vi "Lab Panel V4.85.vi"() -> ()   [LabVIEW 2013] (continued)
                    # "start new test and create test file"
                    n881 = stacked-sequence {
                      seq-local: [w1542 _ _ _ _] -> [_ w1566 _ _ _]
                      tunnel: w1541 -> [w1547 _ _ _ _]
                      tunnel: w1540 -> [w1543 _ _ _ _]
                      tunnel: w1539 -> [w1557 _ _ _ _]
                      tunnel: w1538 -> [w1550 _ _ _ _]
                      tunnel: w1537 -> [w1545 _ _ _ _]
                      tunnel: [_ w1561 _ _ _] -> w1536
                      tunnel: w1535 -> [_ _ _ w1586 _]
                      tunnel: w1534 -> [_ _ _ w1585 _]
                      tunnel: w1533 -> [_ _ _ w1584 _]
                      frame #0 {
                        w1544 = "\\"
                        n882 = local read "SET LAB05-1"() -> (w1552:T5)
                        n883 = case shown="\"CYCLE TEST\"" w1557 {
                          tunnel: ["L05-1-CHART TEST-" "L05-1-CYCLE TEST-" "L05-1-T-RISE TEST-"] -> w1553
                          frame "CHART TEST", Default {
                          }
                          frame "CYCLE TEST" {
                          }
                          frame "T-RISE TEST" {
                          }
                        }
                        n884 = Unbundle(w1552) -> ("DESCRIPTION"=w1551:string)  [unwired: 4 out]
                        n885 = Concatenate Strings(w1547, "\\", w1545, w1544, w1543, w1544) -> (w1554:string)
                        n886 = String To Path(string=w1554) -> (path=w1556:path)
                        n887 = Concatenate Strings(w1554, w1553, w1551, "-", w1550, ".tdms") -> (w1542:string)
                        n888 = Create Folder(path (use dialog)=w1556) -> (error out=w1555:errorcluster)  [unwired: 2 in, 2 out]
                        n889 = global write "Global 1.vi" "LAB05-1 FILE"(w1542) -> ()
                        n890 = call <vilib>:"Clear Errors.vi"("error in (no error)"=w1555) -> ()  [unwired: 6 in, 1 out]
                      }
                      frame #1 {
                        (unwired) FALSE
                        n891 = String To Path(string=w1566) -> (path=w1562:path)
                        n892 = TDMS Open(6:FALSE, 10:T18."create or replace" ("operation (0:open)"), 11:w1562) -> (0:w1561:errorcluster, 3:→"TDMS LAB05-1":refnum<k34>)  [unwired: 4 in]
                      }
                      frame #2 {
                        n893 = local read "SET LAB05-1"() -> (w1572:T5)
                        n894 = local read "TDMS LAB05-1"() -> (w1583:refnum<k34>)
                        n895 = Build Array("Testers Name", "Description", "Set Test Cycles", "T-Rise minutes", "T-Rise Deg C") -> (w1573:string[])
                        n896 = Unbundle(w1572) -> ("NAME"=w1571:string, "DESCRIPTION"=w1570:string, "CYCLES"=w1569:dbl, "T-RISE mins"=w1568:dbl, "T-RISE deg C"=w1567:dbl)
                        n897 = Number To Decimal String(number=w1569) -> (decimal integer string=w1582:string)  [unwired: 1 in]
                        n898 = Number To Decimal String(number=w1568) -> (decimal integer string=w1581:string)  [unwired: 1 in]
                        n899 = Number To Decimal String(number=w1567) -> (decimal integer string=w1580:string)  [unwired: 1 in]
                        n900 = Build Array(w1571, w1570, w1582, w1581, w1580) -> (w1579:string[])
                        n901 = TDMS Set Properties(5:w1579, 7:w1573, 11:w1583) -> ()  [unwired: 3 in, 4 out]
                      }
                      frame #3 {
                        n902 = local read "DISP LAB05-1"() -> (w1588:T4)
                        n903 = Concatenate Strings("LAB05-1  ", w1586) -> (w1589:string)
                        n904 = Two Button Dialog(message=w1589, 1:w1584, 2:w1585) -> (T button?=w1591:bool)
                        n905 = case shown="True" w1591 {
                          tunnel: w1588 -> [w1598 w1599]
                          tunnel: [w1598 w1599] -> w1595
                          tunnel: [w1597 w1600] -> w1594
                          tunnel: [w1596 w1600] -> w1593
                          frame False {
                            n906 = Unbundle(w1598) -> ("CYCLE"=w1597:dbl, "MINS"=w1596:dbl)  [unwired: 1 out]
                          }
                          frame True {
                            w1600 = 0.0
                          }
                        }
                        n907 = Bundle(cluster=w1595, "CYCLE"=w1594, "MINS"=w1593, "STATUS"="RUN") -> (w1587:T4)
                        n908 = local write "DISP LAB05-1"(w1587) -> ()
                      }
                      frame #4 {
                        n909 = local read "SIG LAB05-1"() -> (w1603:T2)
                        n910 = local read "TEMP START LAB05-1"() -> (w1605:cluster{"TL":dbl, "TN":dbl})
                        n911 = Unbundle(w1603) -> ("Tmp Live"=w1602:dbl, "Tmp Neut"=w1601:dbl)  [unwired: 3 out]
                        n912 = Bundle(cluster=w1605, "TL"=w1602, "TN"=w1601) -> (w1604:cluster{"TL":dbl, "TN":dbl})
                        n913 = local write "TEMP START LAB05-1"(w1604) -> ()
                      }
                    }
                  }
                }
              }
              event "RUN LAB05-2": Value Change {
                n914 = event-data() -> ("NewVal"=w1609:bool)  [unwired: 1 in, 5 out]
                n915 = local write "run lab05-2"(w1609) -> ()
                n916 = case shown="True" w1609 {
                  tunnel: w1615 -> [_ w1651]
                  tunnel: w1614 -> [_ w1650]
                  tunnel: w1612 -> [w1617 w1649]
                  tunnel: w1613 -> [_ w1648]
                  tunnel: w1611 -> [_ w1647]
                  tunnel: [w1616 w1646] -> w1610
                  tunnel: w1608 -> [_ w1645]
                  tunnel: w1607 -> [_ w1644]
                  tunnel: w1606 -> [_ w1643]
                  frame False {
                    # "stop test"
                    n917 = stacked-sequence {
                      tunnel: w1617 -> [w1626 _]
                      tunnel: [w1618 _] -> w1616
                      frame #0 {
                        n918 = local read "DISP LAB05-2"() -> (w1625:T4)
                        n919 = Unbundle(w1625) -> ("CYCLE"=w1623:dbl, "MINS"=w1624:dbl)  [unwired: 1 out]
                        n920 = case shown="\"CYCLE TEST\"" w1626 {
                          tunnel: w1624 -> [_ _ w1633]
                          tunnel: w1623 -> [w1631 w1632 _]
                          tunnel: [w1631 w1632 w1633] -> w1622
                          frame "CHART TEST", Default {
                          }
                          frame "CYCLE TEST" {
                          }
                          frame "T-RISE TEST" {
                          }
                        }
                        n921 = local read "TDMS LAB05-2"() -> (w1630:refnum<k34>)
                        n922 = Build Array("STOPPED") -> (w1627:string[])
                        n923 = Build Array(w1622) -> (w1621:dbl[])
                        n924 = TDMS Write(0:w1630, 5:"TEST RESULT", 7:w1627, 9:w1621) -> (4:w1619:refnum<k34>, 15:w1620:errorcluster)  [unwired: 2 in, 2 out]
                        n925 = TDMS Close(8:w1620, 11:w1619) -> (0:w1618:errorcluster)  [unwired: 1 out]
                      }
                      frame #1 {
                        n926 = local read "DISP LAB05-2"() -> (w1637:T4)
                        n927 = stacked-sequence {
                          tunnel: "LAB05-2" -> [w1639 w1641]
                          frame #0 {
                            n928 = call "sub vi - defrag tdms v1.vi"("panel id"=w1639) -> ("error out"=w1638:errorcluster)  [unwired: 10 in]
                            n929 = local write "data file error"(w1638) -> ()
                          }
                          frame #1 {
                            n930 = local write "RESULT LAB05-2"(FALSE) -> ()
                            n931 = call "Save data file to network drive v2.vi"("panel id"=w1641) -> ("network file save error"=w1640:errorcluster)  [unwired: 9 in, 1 out]
                            n932 = local write "data file error"(w1640) -> ()
                          }
                        }
                        n933 = Bundle(cluster=w1637, "STATUS"="STOP") -> (w1635:T4)  [unwired: 2 in]
                        n934 = local write "DISP LAB05-2"(w1635) -> ()
                      }
                    }
                  }
                  frame True {
                    # "start new test and create test file"
                    n935 = stacked-sequence {
                      seq-local: [w1652 _ _ _ _] -> [_ w1676 _ _ _]
                      tunnel: w1651 -> [w1657 _ _ _ _]
                      tunnel: w1650 -> [w1653 _ _ _ _]
                      tunnel: w1649 -> [w1667 _ _ _ _]
                      tunnel: w1648 -> [w1660 _ _ _ _]
                      tunnel: w1647 -> [w1655 _ _ _ _]
                      tunnel: [_ w1671 _ _ _] -> w1646
                      tunnel: w1645 -> [_ _ _ w1696 _]
                      tunnel: w1644 -> [_ _ _ w1695 _]
                      tunnel: w1643 -> [_ _ _ w1694 _]
                      frame #0 {
                        w1654 = "\\"
                        n936 = local read "SET LAB05-2"() -> (w1662:T5)
                        n937 = case shown="\"CYCLE TEST\"" w1667 {
                          tunnel: ["L05-2-CHART TEST-" "L05-2-CYCLE TEST-" "L05-2-T-RISE TEST-"] -> w1663
                          frame "CHART TEST", Default {
                          }
                          frame "CYCLE TEST" {
                          }
                          frame "T-RISE TEST" {
                          }
                        }
                        n938 = Unbundle(w1662) -> ("DESCRIPTION"=w1661:string)  [unwired: 4 out]
                        n939 = Concatenate Strings(w1657, "\\", w1655, w1654, w1653, w1654) -> (w1664:string)
                        n940 = String To Path(string=w1664) -> (path=w1666:path)
                        n941 = Concatenate Strings(w1664, w1663, w1661, "-", w1660, ".tdms") -> (w1652:string)
                        n942 = Create Folder(path (use dialog)=w1666) -> (error out=w1665:errorcluster)  [unwired: 2 in, 2 out]
                        n943 = global write "Global 1.vi" "LAB05-2 FILE"(w1652) -> ()
                        n944 = call <vilib>:"Clear Errors.vi"("error in (no error)"=w1665) -> ()  [unwired: 6 in, 1 out]
                      }
                      frame #1 {
                        (unwired) FALSE
                        n945 = String To Path(string=w1676) -> (path=w1672:path)
                        n946 = TDMS Open(6:FALSE, 10:T18."create or replace" ("operation (0:open)"), 11:w1672) -> (0:w1671:errorcluster, 3:→"TDMS LAB05-2":refnum<k34>)  [unwired: 4 in]
                      }
                      frame #2 {
                        n947 = local read "SET LAB05-2"() -> (w1682:T5)
                        n948 = local read "TDMS LAB05-2"() -> (w1693:refnum<k34>)
                        n949 = Build Array("Testers Name", "Description", "Set Test Cycles", "T-Rise minutes", "T-Rise Deg C") -> (w1683:string[])
                        n950 = Unbundle(w1682) -> ("NAME"=w1681:string, "DESCRIPTION"=w1680:string, "CYCLES"=w1679:dbl, "T-RISE mins"=w1678:dbl, "T-RISE deg C"=w1677:dbl)
                        n951 = Number To Decimal String(number=w1679) -> (decimal integer string=w1692:string)  [unwired: 1 in]
                        n952 = Number To Decimal String(number=w1678) -> (decimal integer string=w1691:string)  [unwired: 1 in]
                        n953 = Number To Decimal String(number=w1677) -> (decimal integer string=w1690:string)  [unwired: 1 in]
                        n954 = Build Array(w1681, w1680, w1692, w1691, w1690) -> (w1689:string[])
                        n955 = TDMS Set Properties(5:w1689, 7:w1683, 11:w1693) -> ()  [unwired: 3 in, 4 out]
                      }
                      frame #3 {
                        n956 = local read "DISP LAB05-2"() -> (w1698:T4)
                        n957 = Concatenate Strings("LAB05-2  ", w1696) -> (w1699:string)
                        n958 = Two Button Dialog(message=w1699, 1:w1694, 2:w1695) -> (T button?=w1701:bool)
                        n959 = case shown="True" w1701 {
                          tunnel: w1698 -> [w1708 w1709]
                          tunnel: [w1708 w1709] -> w1705
                          tunnel: [w1707 w1710] -> w1704
                          tunnel: [w1706 w1710] -> w1703
                          frame False {
                            n960 = Unbundle(w1708) -> ("CYCLE"=w1707:dbl, "MINS"=w1706:dbl)  [unwired: 1 out]
                          }
                          frame True {
                            w1710 = 0.0
                          }
                        }
                        n961 = Bundle(cluster=w1705, "CYCLE"=w1704, "MINS"=w1703, "STATUS"="RUN") -> (w1697:T4)
                        n962 = local write "DISP LAB05-2"(w1697) -> ()
                      }
                      frame #4 {
                        n963 = local read "SIG LAB05-2"() -> (w1713:T2)
                        n964 = local read "TEMP START LAB05-2"() -> (w1715:cluster{"TL":dbl, "TN":dbl})
                        n965 = Unbundle(w1713) -> ("Tmp Live"=w1712:dbl, "Tmp Neut"=w1711:dbl)  [unwired: 3 out]
                        n966 = Bundle(cluster=w1715, "TL"=w1712, "TN"=w1711) -> (w1714:cluster{"TL":dbl, "TN":dbl})
                        n967 = local write "TEMP START LAB05-2"(w1714) -> ()
                      }
                    }
                  }
                }
              }
            }
            n968 = local write "data file error"(w587) -> ()
          }
          frame #4 {
            # "check if test cycles reached for cycle tests, if so then test pass"
            n969 = stacked-sequence {
              tunnel: w1735 -> [_ _ _ _ _ _ _ _ _ _]
              tunnel: w1734 -> [_ _ _ _ _ _ _ _ _ _]
              tunnel: w1733 -> [_ _ _ _ _ _ _ _ _ _]
              tunnel: w1732 -> [_ _ _ _ _ _ _ _ _ _]
              tunnel: w1731 -> [_ _ _ _ _ _ _ _ _ _]
              tunnel: w1730 -> [_ _ _ _ _ _ _ _ _ _]
              tunnel: w1729 -> [_ _ _ _ _ _ _ _ _ _]
              tunnel: w1728 -> [_ _ _ _ _ _ _ _ _ _]
              tunnel: w1727 -> [_ _ _ _ _ _ _ _ _ _]
              tunnel: w1726 -> [_ _ _ _ _ _ _ _ _ _]
              tunnel: w1725 -> [w1741 _ _ _ _ _ _ _ _ _]
              tunnel: w1724 -> [_ w1776 _ _ _ _ _ _ _ _]
              tunnel: w1723 -> [_ _ w1816 _ _ _ _ _ _ _]
              tunnel: w1722 -> [_ _ _ w1856 _ _ _ _ _ _]
              tunnel: w1721 -> [_ _ _ _ w1896 _ _ _ _ _]
              tunnel: w1720 -> [_ _ _ _ _ w1936 _ _ _ _]
              tunnel: w1719 -> [_ _ _ _ _ _ w1976 _ _ _]
              tunnel: w1718 -> [_ _ _ _ _ _ _ w2016 _ _]
              tunnel: w1717 -> [_ _ _ _ _ _ _ _ w2056 _]
              tunnel: w1716 -> [_ _ _ _ _ _ _ _ _ w2096]
              frame #0 {
                # "LAB01-1"
                n970 = Less?(x=w1741, y=2) -> (x < y?=w1739:bool)
                n971 = local read "DISP LAB01-1"() -> (w1742:T4)
                n972 = Unbundle(w1742) -> ("STATUS"=w1736:string)  [unwired: 2 out]
                n973 = Equal?(x=w1736, y="RUN") -> (x = y?=w1738:bool)
                n974 = And(x=w1738, y=w1739) -> (x .and. y?=w1737:bool)
                n975 = case shown="True" w1737 {
                  tunnel: w1742 -> [_ w1747]
                  tunnel: w1741 -> [_ w1751]
                  frame False {
                  }
                  frame True {
                    n976 = local read "SET LAB01-1"() -> (w1753:T5)
                    n977 = local read "TDMS LAB01-1"() -> (w1746:refnum<k34>)
                    n978 = Unbundle(w1753) -> ("CYCLES"=w1744:dbl, "T-RISE mins"=w1750:dbl)  [unwired: 3 out]
                    n979 = case shown="\"CYCLE TEST\"" w1751 {
                      tunnel: w1750 -> [_ _ w1760]
                      tunnel: [w1755 w1757 w1760] -> w1749
                      tunnel: w1744 -> [w1755 w1757 _]
                      tunnel: ["CHART PASS" "CYCLE PASS" "T-RISE PASS"] -> w1748
                      frame "CHART TEST", Default {
                      }
                      frame "CYCLE TEST" {
                      }
                      frame "T-RISE TEST" {
                      }
                    }
                    n980 = Unbundle(w1747) -> ("CYCLE"=w1752:dbl)  [unwired: 2 out]
                    n981 = Increment(x=w1744) -> (x+1=w1745:dbl)
                    n982 = Greater Or Equal?(x=w1752, y=w1745) -> (x >= y?=w1754:bool)
                    n983 = case shown="True" w1754 {
                      tunnel: w1749 -> [w1764 _]
                      tunnel: w1748 -> [w1763 _]
                      tunnel: w1747 -> [w1762 _]
                      tunnel: w1746 -> [w1761 _]
                      frame True {
                        n984 = stacked-sequence {
                          tunnel: w1764 -> [w1768 _]
                          tunnel: w1763 -> [w1766 w1772]
                          tunnel: w1762 -> [_ w1775]
                          tunnel: w1761 -> [w1765 _]
                          frame #0 {
                            n985 = Build Array(w1766) -> (w1769:string[])
                            n986 = Build Array(w1768) -> (w1767:dbl[])
                            n987 = TDMS Write(0:w1765, 5:"TEST PASS", 7:w1769, 9:w1767) -> (15:w1771:errorcluster)  [unwired: 2 in, 3 out]
                            n988 = local write "data file error"(w1771) -> ()
                          }
                          frame #1 {
                            n989 = Bundle(cluster=w1775, "STATUS"=w1772) -> (w1773:T4)  [unwired: 2 in]
                            n990 = local write "RESULT LAB01-1"(TRUE) -> ()
                            n991 = local write "DISP LAB01-1"(w1773) -> ()
                          }
                        }
                      }
                      frame False {
                      }
                    }
                  }
                }
              }
              frame #1 {
                # "LAB01-2"
                n992 = Less?(x=w1776, y=2) -> (x < y?=w1779:bool)
                n993 = local read "DISP LAB01-2"() -> (w1781:T4)
                n994 = Unbundle(w1781) -> ("STATUS"=w1782:string)  [unwired: 2 out]
                n995 = Equal?(x=w1782, y="RUN") -> (x = y?=w1778:bool)
                n996 = And(x=w1778, y=w1779) -> (x .and. y?=w1777:bool)
                n997 = case shown="True" w1777 {
                  tunnel: w1781 -> [_ w1787]
                  tunnel: w1776 -> [_ w1791]
                  frame False {
                  }
                  frame True {
                    n998 = local read "SET LAB01-2"() -> (w1793:T5)
                    n999 = local read "TDMS LAB01-2"() -> (w1786:refnum<k34>)
                    n1000 = Unbundle(w1793) -> ("CYCLES"=w1784:dbl, "T-RISE mins"=w1790:dbl)  [unwired: 3 out]
                    n1001 = case shown="\"T-RISE TEST\"" w1791 {
                      tunnel: w1790 -> [_ _ w1800]
                      tunnel: [w1795 w1797 w1800] -> w1789
                      tunnel: w1784 -> [w1795 w1797 _]
                      tunnel: ["CHART PASS" "CYCLE PASS" "T-RISE PASS"] -> w1788
                      frame "CHART TEST", Default {
                      }
                      frame "CYCLE TEST" {
                      }
                      frame "T-RISE TEST" {
                      }
                    }
                    n1002 = Unbundle(w1787) -> ("CYCLE"=w1792:dbl)  [unwired: 2 out]
                    n1003 = Increment(x=w1784) -> (x+1=w1785:dbl)
                    n1004 = Greater Or Equal?(x=w1792, y=w1785) -> (x >= y?=w1794:bool)
                    n1005 = case shown="True" w1794 {
                      tunnel: w1789 -> [w1804 _]
                      tunnel: w1788 -> [w1803 _]
                      tunnel: w1787 -> [w1802 _]
                      tunnel: w1786 -> [w1801 _]
                      frame True {
                        n1006 = stacked-sequence {
                          tunnel: w1804 -> [w1808 _]
                          tunnel: w1803 -> [w1806 w1812]
                          tunnel: w1802 -> [_ w1815]
                          tunnel: w1801 -> [w1805 _]
                          frame #0 {
                            n1007 = Build Array(w1806) -> (w1809:string[])
                            n1008 = Build Array(w1808) -> (w1807:dbl[])
                            n1009 = TDMS Write(0:w1805, 5:"TEST PASS", 7:w1809, 9:w1807) -> (15:w1811:errorcluster)  [unwired: 2 in, 3 out]
                            n1010 = local write "data file error"(w1811) -> ()
                          }
                          frame #1 {
                            n1011 = Bundle(cluster=w1815, "STATUS"=w1812) -> (w1813:T4)  [unwired: 2 in]
                            n1012 = local write "RESULT LAB01-2"(TRUE) -> ()
                            n1013 = local write "DISP LAB01-2"(w1813) -> ()
                          }
                        }
                      }
                      frame False {
                      }
                    }
                  }
                }
              }
              frame #2 {
                # "LAB02-1"
                n1014 = Less?(x=w1816, y=2) -> (x < y?=w1819:bool)
                n1015 = local read "DISP LAB02-1"() -> (w1821:T4)
                n1016 = Unbundle(w1821) -> ("STATUS"=w1822:string)  [unwired: 2 out]
                n1017 = Equal?(x=w1822, y="RUN") -> (x = y?=w1818:bool)
                n1018 = And(x=w1818, y=w1819) -> (x .and. y?=w1817:bool)
                n1019 = case shown="True" w1817 {
                  tunnel: w1821 -> [_ w1827]
                  tunnel: w1816 -> [_ w1831]
                  frame False {
                  }
                  frame True {
                    n1020 = local read "SET LAB02-1"() -> (w1833:T5)
                    n1021 = local read "TDMS LAB02-1"() -> (w1826:refnum<k34>)
                    n1022 = Unbundle(w1827) -> ("CYCLE"=w1832:dbl)  [unwired: 2 out]
                    n1023 = Unbundle(w1833) -> ("CYCLES"=w1824:dbl, "T-RISE mins"=w1830:dbl)  [unwired: 3 out]
                    n1024 = case shown="\"T-RISE TEST\"" w1831 {
                      tunnel: w1830 -> [_ _ w1840]
                      tunnel: [w1835 w1837 w1840] -> w1829
                      tunnel: w1824 -> [w1835 w1837 _]
                      tunnel: ["CHART PASS" "CYCLE PASS" "T-RISE PASS"] -> w1828
                      frame "CHART TEST", Default {
                      }
                      frame "CYCLE TEST" {
                      }
                      frame "T-RISE TEST" {
                      }
                    }
                    n1025 = Increment(x=w1824) -> (x+1=w1825:dbl)
                    n1026 = Greater Or Equal?(x=w1832, y=w1825) -> (x >= y?=w1834:bool)
                    n1027 = case shown="True" w1834 {
                      tunnel: w1829 -> [w1844 _]
                      tunnel: w1828 -> [w1843 _]
                      tunnel: w1827 -> [w1842 _]
                      tunnel: w1826 -> [w1841 _]
                      frame True {
                        n1028 = stacked-sequence {
                          tunnel: w1844 -> [w1848 _]
                          tunnel: w1843 -> [w1846 w1852]
                          tunnel: w1842 -> [_ w1855]
                          tunnel: w1841 -> [w1845 _]
                          frame #0 {
                            n1029 = Build Array(w1846) -> (w1849:string[])
                            n1030 = Build Array(w1848) -> (w1847:dbl[])
                            n1031 = TDMS Write(0:w1845, 5:"TEST PASS", 7:w1849, 9:w1847) -> (15:w1851:errorcluster)  [unwired: 2 in, 3 out]
                            n1032 = local write "data file error"(w1851) -> ()
                          }
                          frame #1 {
                            n1033 = Bundle(cluster=w1855, "STATUS"=w1852) -> (w1853:T4)  [unwired: 2 in]
                            n1034 = local write "RESULT LAB02-1"(TRUE) -> ()
                            n1035 = local write "DISP LAB02-1"(w1853) -> ()
                          }
                        }
                      }
                      frame False {
                      }
                    }
                  }
                }
              }
              frame #3 {
                # "LAB02-2"
                n1036 = Less?(x=w1856, y=2) -> (x < y?=w1859:bool)
                n1037 = local read "DISP LAB02-2"() -> (w1861:T4)
                n1038 = Unbundle(w1861) -> ("STATUS"=w1862:string)  [unwired: 2 out]
                n1039 = Equal?(x=w1862, y="RUN") -> (x = y?=w1858:bool)
                n1040 = And(x=w1858, y=w1859) -> (x .and. y?=w1857:bool)
                n1041 = case shown="True" w1857 {
                  tunnel: w1861 -> [_ w1867]
                  tunnel: w1856 -> [_ w1871]
                  frame False {
                  }
                  frame True {
                    n1042 = local read "SET LAB02-2"() -> (w1873:T5)
                    n1043 = local read "TDMS LAB02-2"() -> (w1866:refnum<k34>)
                    n1044 = Unbundle(w1867) -> ("CYCLE"=w1872:dbl)  [unwired: 2 out]
                    n1045 = Unbundle(w1873) -> ("CYCLES"=w1864:dbl, "T-RISE mins"=w1870:dbl)  [unwired: 3 out]
                    n1046 = case shown="\"T-RISE TEST\"" w1871 {
                      tunnel: w1870 -> [_ _ w1880]
                      tunnel: [w1875 w1877 w1880] -> w1869
                      tunnel: w1864 -> [w1875 w1877 _]
                      tunnel: ["CHART PASS" "CYCLE PASS" "T-RISE PASS"] -> w1868
                      frame "CHART TEST", Default {
                      }
                      frame "CYCLE TEST" {
                      }
                      frame "T-RISE TEST" {
                      }
                    }
                    n1047 = Increment(x=w1864) -> (x+1=w1865:dbl)
                    n1048 = Greater Or Equal?(x=w1872, y=w1865) -> (x >= y?=w1874:bool)
                    n1049 = case shown="True" w1874 {
                      tunnel: w1869 -> [w1884 _]
                      tunnel: w1868 -> [w1883 _]
                      tunnel: w1867 -> [w1882 _]
                      tunnel: w1866 -> [w1881 _]
                      frame True {
                        n1050 = stacked-sequence {
                          tunnel: w1884 -> [w1888 _]
                          tunnel: w1883 -> [w1886 w1892]
                          tunnel: w1882 -> [_ w1895]
                          tunnel: w1881 -> [w1885 _]
                          frame #0 {
                            n1051 = Build Array(w1886) -> (w1889:string[])
                            n1052 = Build Array(w1888) -> (w1887:dbl[])
                            n1053 = TDMS Write(0:w1885, 5:"TEST PASS", 7:w1889, 9:w1887) -> (15:w1891:errorcluster)  [unwired: 2 in, 3 out]
                            n1054 = local write "data file error"(w1891) -> ()
                          }
                          frame #1 {
                            n1055 = Bundle(cluster=w1895, "STATUS"=w1892) -> (w1893:T4)  [unwired: 2 in]
                            n1056 = local write "RESULT LAB02-2"(TRUE) -> ()
                            n1057 = local write "DISP LAB02-2"(w1893) -> ()
                          }
                        }
                      }
                      frame False {
                      }
                    }
                  }
                }
              }
              frame #4 {
                # "LAB03-1"
                n1058 = Less?(x=w1896, y=2) -> (x < y?=w1899:bool)
                n1059 = local read "DISP LAB03-1"() -> (w1901:T4)
                n1060 = Unbundle(w1901) -> ("STATUS"=w1902:string)  [unwired: 2 out]
                n1061 = Equal?(x=w1902, y="RUN") -> (x = y?=w1898:bool)
                n1062 = And(x=w1898, y=w1899) -> (x .and. y?=w1897:bool)
                n1063 = case shown="True" w1897 {
                  tunnel: w1901 -> [_ w1907]
                  tunnel: w1896 -> [_ w1911]
                  frame False {
                  }
                  frame True {
                    n1064 = local read "SET LAB03-1"() -> (w1913:T5)
                    n1065 = local read "TDMS LAB03-1"() -> (w1906:refnum<k34>)
                    n1066 = Unbundle(w1907) -> ("CYCLE"=w1912:dbl)  [unwired: 2 out]
                    n1067 = Unbundle(w1913) -> ("CYCLES"=w1904:dbl, "T-RISE mins"=w1910:dbl)  [unwired: 3 out]
                    n1068 = case shown="\"T-RISE TEST\"" w1911 {
                      tunnel: w1910 -> [_ _ w1920]
                      tunnel: [w1915 w1917 w1920] -> w1909
                      tunnel: w1904 -> [w1915 w1917 _]
                      tunnel: ["CHART PASS" "CYCLE PASS" "T-RISE PASS"] -> w1908
                      frame "CHART TEST", Default {
                      }
                      frame "CYCLE TEST" {
                      }
                      frame "T-RISE TEST" {
                      }
                    }
                    n1069 = Increment(x=w1904) -> (x+1=w1905:dbl)
                    n1070 = Greater Or Equal?(x=w1912, y=w1905) -> (x >= y?=w1914:bool)
                    n1071 = case shown="True" w1914 {
                      tunnel: w1909 -> [w1924 _]
                      tunnel: w1908 -> [w1923 _]
                      tunnel: w1907 -> [w1922 _]
                      tunnel: w1906 -> [w1921 _]
                      frame True {
                        n1072 = stacked-sequence {
                          tunnel: w1924 -> [w1928 _]
                          tunnel: w1923 -> [w1926 w1932]
                          tunnel: w1922 -> [_ w1935]
                          tunnel: w1921 -> [w1925 _]
                          frame #0 {
                            n1073 = Build Array(w1926) -> (w1929:string[])
                            n1074 = Build Array(w1928) -> (w1927:dbl[])
                            n1075 = TDMS Write(0:w1925, 5:"TEST PASS", 7:w1929, 9:w1927) -> (15:w1931:errorcluster)  [unwired: 2 in, 3 out]
                            n1076 = local write "data file error"(w1931) -> ()
                          }
                          frame #1 {
                            n1077 = Bundle(cluster=w1935, "STATUS"=w1932) -> (w1933:T4)  [unwired: 2 in]
                            n1078 = local write "RESULT LAB03-1"(TRUE) -> ()
                            n1079 = local write "DISP LAB03-1"(w1933) -> ()
                          }
                        }
                      }
                      frame False {
                      }
                    }
                  }
                }
              }
              frame #5 {
                # "LAB03-2"
                n1080 = Less?(x=w1936, y=2) -> (x < y?=w1939:bool)
                n1081 = local read "DISP LAB03-2"() -> (w1941:T4)
                n1082 = Unbundle(w1941) -> ("STATUS"=w1942:string)  [unwired: 2 out]
                n1083 = Equal?(x=w1942, y="RUN") -> (x = y?=w1938:bool)
                n1084 = And(x=w1938, y=w1939) -> (x .and. y?=w1937:bool)
                n1085 = case shown="True" w1937 {
                  tunnel: w1941 -> [_ w1947]
                  tunnel: w1936 -> [_ w1951]
                  frame False {
                  }
                  frame True {
                    n1086 = local read "SET LAB03-2"() -> (w1953:T5)
                    n1087 = local read "TDMS LAB03-2"() -> (w1946:refnum<k34>)
                    n1088 = Unbundle(w1947) -> ("CYCLE"=w1952:dbl)  [unwired: 2 out]
                    n1089 = Unbundle(w1953) -> ("CYCLES"=w1944:dbl, "T-RISE mins"=w1950:dbl)  [unwired: 3 out]
                    n1090 = case shown="\"T-RISE TEST\"" w1951 {
                      tunnel: w1950 -> [_ _ w1960]
                      tunnel: [w1955 w1957 w1960] -> w1949
                      tunnel: w1944 -> [w1955 w1957 _]
                      tunnel: ["CHART PASS" "CYCLE PASS" "T-RISE PASS"] -> w1948
                      frame "CHART TEST", Default {
                      }
                      frame "CYCLE TEST" {
                      }
                      frame "T-RISE TEST" {
                      }
                    }
                    n1091 = Increment(x=w1944) -> (x+1=w1945:dbl)
                    n1092 = Greater Or Equal?(x=w1952, y=w1945) -> (x >= y?=w1954:bool)
                    n1093 = case shown="True" w1954 {
                      tunnel: w1949 -> [w1964 _]
                      tunnel: w1948 -> [w1963 _]
                      tunnel: w1947 -> [w1962 _]
                      tunnel: w1946 -> [w1961 _]
                      frame True {
                        n1094 = stacked-sequence {
                          tunnel: w1964 -> [w1968 _]
                          tunnel: w1963 -> [w1966 w1972]
                          tunnel: w1962 -> [_ w1975]
                          tunnel: w1961 -> [w1965 _]
                          frame #0 {
                            n1095 = Build Array(w1966) -> (w1969:string[])
                            n1096 = Build Array(w1968) -> (w1967:dbl[])
                            n1097 = TDMS Write(0:w1965, 5:"TEST PASS", 7:w1969, 9:w1967) -> (15:w1971:errorcluster)  [unwired: 2 in, 3 out]
                            n1098 = local write "data file error"(w1971) -> ()
                          }
                          frame #1 {
                            n1099 = Bundle(cluster=w1975, "STATUS"=w1972) -> (w1973:T4)  [unwired: 2 in]
                            n1100 = local write "RESULT LAB03-2"(TRUE) -> ()
                            n1101 = local write "DISP LAB03-2"(w1973) -> ()
                          }
                        }
                      }
                      frame False {
                      }
                    }
                  }
                }
              }
              frame #6 {
                # "LAB04-1"
                n1102 = Less?(x=w1976, y=2) -> (x < y?=w1979:bool)
                n1103 = local read "DISP LAB04-1"() -> (w1981:T4)
                n1104 = Unbundle(w1981) -> ("STATUS"=w1982:string)  [unwired: 2 out]
                n1105 = Equal?(x=w1982, y="RUN") -> (x = y?=w1978:bool)
                n1106 = And(x=w1978, y=w1979) -> (x .and. y?=w1977:bool)
                n1107 = case shown="True" w1977 {
                  tunnel: w1981 -> [_ w1987]
                  tunnel: w1976 -> [_ w1991]
                  frame False {
                  }
                  frame True {
                    n1108 = local read "SET LAB04-1"() -> (w1993:T5)
                    n1109 = local read "TDMS LAB04-1"() -> (w1986:refnum<k34>)
                    n1110 = Unbundle(w1987) -> ("CYCLE"=w1992:dbl)  [unwired: 2 out]
                    n1111 = Unbundle(w1993) -> ("CYCLES"=w1984:dbl, "T-RISE mins"=w1990:dbl)  [unwired: 3 out]
                    n1112 = case shown="\"T-RISE TEST\"" w1991 {
                      tunnel: w1990 -> [_ _ w2000]
                      tunnel: [w1995 w1997 w2000] -> w1989
                      tunnel: w1984 -> [w1995 w1997 _]
                      tunnel: ["CHART PASS" "CYCLE PASS" "T-RISE PASS"] -> w1988
                      frame "CHART TEST", Default {
                      }
                      frame "CYCLE TEST" {
                      }
                      frame "T-RISE TEST" {
                      }
                    }
                    n1113 = Increment(x=w1984) -> (x+1=w1985:dbl)
                    n1114 = Greater Or Equal?(x=w1992, y=w1985) -> (x >= y?=w1994:bool)
                    n1115 = case shown="True" w1994 {
                      tunnel: w1989 -> [w2004 _]
                      tunnel: w1988 -> [w2003 _]
                      tunnel: w1987 -> [w2002 _]
                      tunnel: w1986 -> [w2001 _]
                      frame True {
                        n1116 = stacked-sequence {
                          tunnel: w2004 -> [w2008 _]
                          tunnel: w2003 -> [w2006 w2012]
                          tunnel: w2002 -> [_ w2015]
                          tunnel: w2001 -> [w2005 _]
                          frame #0 {
                            n1117 = Build Array(w2006) -> (w2009:string[])
                            n1118 = Build Array(w2008) -> (w2007:dbl[])
                            n1119 = TDMS Write(0:w2005, 5:"TEST PASS", 7:w2009, 9:w2007) -> (15:w2011:errorcluster)  [unwired: 2 in, 3 out]
                            n1120 = local write "data file error"(w2011) -> ()
                          }
                          frame #1 {
                            n1121 = Bundle(cluster=w2015, "STATUS"=w2012) -> (w2013:T4)  [unwired: 2 in]
                            n1122 = local write "RESULT LAB04-1"(TRUE) -> ()
                            n1123 = local write "DISP LAB04-1"(w2013) -> ()
                          }
                        }
                      }
                      frame False {
                      }
                    }
                  }
                }
              }
              frame #7 {
                # "LAB04-2"
                n1124 = Less?(x=w2016, y=2) -> (x < y?=w2019:bool)
                n1125 = local read "DISP LAB04-2"() -> (w2021:T4)
                n1126 = Unbundle(w2021) -> ("STATUS"=w2022:string)  [unwired: 2 out]
                n1127 = Equal?(x=w2022, y="RUN") -> (x = y?=w2018:bool)
                n1128 = And(x=w2018, y=w2019) -> (x .and. y?=w2017:bool)
                n1129 = case shown="True" w2017 {
                  tunnel: w2021 -> [_ w2027]
                  tunnel: w2016 -> [_ w2031]
                  frame False {
                  }
                  frame True {
                    n1130 = local read "SET LAB04-2"() -> (w2033:T5)
                    n1131 = local read "TDMS LAB04-2"() -> (w2026:refnum<k34>)
                    n1132 = Unbundle(w2027) -> ("CYCLE"=w2032:dbl)  [unwired: 2 out]
                    n1133 = Unbundle(w2033) -> ("CYCLES"=w2024:dbl, "T-RISE mins"=w2030:dbl)  [unwired: 3 out]
                    n1134 = case shown="\"T-RISE TEST\"" w2031 {
                      tunnel: w2030 -> [_ _ w2040]
                      tunnel: [w2035 w2037 w2040] -> w2029
                      tunnel: w2024 -> [w2035 w2037 _]
                      tunnel: ["CHART PASS" "CYCLE PASS" "T-RISE PASS"] -> w2028
                      frame "CHART TEST", Default {
                      }
                      frame "CYCLE TEST" {
                      }
                      frame "T-RISE TEST" {
                      }
                    }
                    n1135 = Increment(x=w2024) -> (x+1=w2025:dbl)
                    n1136 = Greater Or Equal?(x=w2032, y=w2025) -> (x >= y?=w2034:bool)
                    n1137 = case shown="True" w2034 {
                      tunnel: w2029 -> [w2044 _]
                      tunnel: w2028 -> [w2043 _]
                      tunnel: w2027 -> [w2042 _]
                      tunnel: w2026 -> [w2041 _]
                      frame True {
                        n1138 = stacked-sequence {
                          tunnel: w2044 -> [w2048 _]
                          tunnel: w2043 -> [w2046 w2052]
                          tunnel: w2042 -> [_ w2055]
                          tunnel: w2041 -> [w2045 _]
                          frame #0 {
                            n1139 = Build Array(w2046) -> (w2049:string[])
                            n1140 = Build Array(w2048) -> (w2047:dbl[])
                            n1141 = TDMS Write(0:w2045, 5:"TEST PASS", 7:w2049, 9:w2047) -> (15:w2051:errorcluster)  [unwired: 2 in, 3 out]
                            n1142 = local write "data file error"(w2051) -> ()
                          }
                          frame #1 {
                            n1143 = Bundle(cluster=w2055, "STATUS"=w2052) -> (w2053:T4)  [unwired: 2 in]
                            n1144 = local write "RESULT LAB04-2"(TRUE) -> ()
                            n1145 = local write "DISP LAB04-2"(w2053) -> ()
                          }
                        }
                      }
                      frame False {
                      }
                    }
                  }
                }
              }
              frame #8 {
                # "LAB05-1"
                n1146 = Less?(x=w2056, y=2) -> (x < y?=w2059:bool)
                n1147 = local read "DISP LAB05-1"() -> (w2061:T4)
                n1148 = Unbundle(w2061) -> ("STATUS"=w2062:string)  [unwired: 2 out]
                n1149 = Equal?(x=w2062, y="RUN") -> (x = y?=w2058:bool)
                n1150 = And(x=w2058, y=w2059) -> (x .and. y?=w2057:bool)
                n1151 = case shown="True" w2057 {
                  tunnel: w2061 -> [_ w2067]
                  tunnel: w2056 -> [_ w2071]
                  frame False {
                  }
                  frame True {
                    n1152 = local read "SET LAB05-1"() -> (w2073:T5)
                    n1153 = local read "TDMS LAB05-1"() -> (w2066:refnum<k34>)
                    n1154 = Unbundle(w2067) -> ("CYCLE"=w2072:dbl)  [unwired: 2 out]
                    n1155 = Unbundle(w2073) -> ("CYCLES"=w2064:dbl, "T-RISE mins"=w2070:dbl)  [unwired: 3 out]
                    n1156 = case shown="\"T-RISE TEST\"" w2071 {
                      tunnel: w2070 -> [_ _ w2080]
                      tunnel: [w2075 w2077 w2080] -> w2069
                      tunnel: w2064 -> [w2075 w2077 _]
                      tunnel: ["CHART PASS" "CYCLE PASS" "T-RISE PASS"] -> w2068
                      frame "CHART TEST", Default {
                      }
                      frame "CYCLE TEST" {
                      }
                      frame "T-RISE TEST" {
                      }
                    }
                    n1157 = Increment(x=w2064) -> (x+1=w2065:dbl)
                    n1158 = Greater Or Equal?(x=w2072, y=w2065) -> (x >= y?=w2074:bool)
                    n1159 = case shown="True" w2074 {
                      tunnel: w2069 -> [w2084 _]
                      tunnel: w2068 -> [w2083 _]
                      tunnel: w2067 -> [w2082 _]
                      tunnel: w2066 -> [w2081 _]
                      frame True {
                        n1160 = stacked-sequence {
                          tunnel: w2084 -> [w2088 _]
                          tunnel: w2083 -> [w2086 w2092]
                          tunnel: w2082 -> [_ w2095]
                          tunnel: w2081 -> [w2085 _]
                          frame #0 {
                            n1161 = Build Array(w2086) -> (w2089:string[])
                            n1162 = Build Array(w2088) -> (w2087:dbl[])
                            n1163 = TDMS Write(0:w2085, 5:"TEST PASS", 7:w2089, 9:w2087) -> (15:w2091:errorcluster)  [unwired: 2 in, 3 out]
                            n1164 = local write "data file error"(w2091) -> ()
                          }
                          frame #1 {
                            n1165 = Bundle(cluster=w2095, "STATUS"=w2092) -> (w2093:T4)  [unwired: 2 in]
                            n1166 = local write "RESULT LAB05-1"(TRUE) -> ()
                            n1167 = local write "DISP LAB05-1"(w2093) -> ()
                          }
                        }
                      }
                      frame False {
                      }
                    }
                  }
                }
              }
              frame #9 {
                # "LAB05-2"
                n1168 = Less?(x=w2096, y=2) -> (x < y?=w2099:bool)
                n1169 = local read "DISP LAB05-2"() -> (w2101:T4)
                n1170 = Unbundle(w2101) -> ("STATUS"=w2102:string)  [unwired: 2 out]
                n1171 = Equal?(x=w2102, y="RUN") -> (x = y?=w2098:bool)
                n1172 = And(x=w2098, y=w2099) -> (x .and. y?=w2097:bool)
                n1173 = case shown="True" w2097 {
                  tunnel: w2101 -> [_ w2107]
                  tunnel: w2096 -> [_ w2111]
                  frame False {
                  }
                  frame True {
                    n1174 = local read "SET LAB05-2"() -> (w2113:T5)
                    n1175 = local read "TDMS LAB05-2"() -> (w2106:refnum<k34>)
                    n1176 = Unbundle(w2107) -> ("CYCLE"=w2112:dbl)  [unwired: 2 out]
                    n1177 = Unbundle(w2113) -> ("CYCLES"=w2104:dbl, "T-RISE mins"=w2110:dbl)  [unwired: 3 out]
                    n1178 = case shown="\"T-RISE TEST\"" w2111 {
                      tunnel: w2110 -> [_ _ w2120]
                      tunnel: [w2115 w2117 w2120] -> w2109
                      tunnel: w2104 -> [w2115 w2117 _]
                      tunnel: ["CHART PASS" "CYCLE PASS" "T-RISE PASS"] -> w2108
                      frame "CHART TEST", Default {
                      }
                      frame "CYCLE TEST" {
                      }
                      frame "T-RISE TEST" {
                      }
                    }
                    n1179 = Increment(x=w2104) -> (x+1=w2105:dbl)
                    n1180 = Greater Or Equal?(x=w2112, y=w2105) -> (x >= y?=w2114:bool)
                    n1181 = case shown="True" w2114 {
                      tunnel: w2109 -> [w2124 _]
                      tunnel: w2108 -> [w2123 _]
                      tunnel: w2107 -> [w2122 _]
                      tunnel: w2106 -> [w2121 _]
                      frame True {
                        n1182 = stacked-sequence {
                          tunnel: w2124 -> [w2128 _]
                          tunnel: w2123 -> [w2126 w2132]
                          tunnel: w2122 -> [_ w2135]
                          tunnel: w2121 -> [w2125 _]
                          frame #0 {
                            n1183 = Build Array(w2126) -> (w2129:string[])
                            n1184 = Build Array(w2128) -> (w2127:dbl[])
                            n1185 = TDMS Write(0:w2125, 5:"TEST PASS", 7:w2129, 9:w2127) -> (15:w2131:errorcluster)  [unwired: 2 in, 3 out]
                            n1186 = local write "data file error"(w2131) -> ()
                          }
                          frame #1 {
                            n1187 = Bundle(cluster=w2135, "STATUS"=w2132) -> (w2133:T4)  [unwired: 2 in]
                            n1188 = local write "RESULT LAB05-2"(TRUE) -> ()
                            n1189 = local write "DISP LAB05-2"(w2133) -> ()
                          }
                        }
                      }
                      frame False {
                      }
                    }
                  }
                }
              }
            }
          }
          frame #5 {
            # "check if test cycles reached for temperature rise test"
            n1190 = stacked-sequence {
              tunnel: w2165 -> [_ _ _ _ _ _ _ _ _ _]
              tunnel: w2164 -> [_ _ _ _ _ _ _ _ _ _]
              tunnel: w2163 -> [_ _ _ _ _ _ _ _ _ _]
              tunnel: w2162 -> [_ _ _ _ _ _ _ _ _ _]
              tunnel: w2161 -> [_ _ _ _ _ _ _ _ _ _]
              tunnel: w2160 -> [_ _ _ _ _ _ _ _ _ _]
              tunnel: w2159 -> [_ _ _ _ _ _ _ _ _ _]
              tunnel: w2158 -> [_ _ _ _ _ _ _ _ _ _]
              tunnel: w2157 -> [_ _ _ _ _ _ _ _ _ _]
              tunnel: w2156 -> [_ _ _ _ _ _ _ _ _ _]
              tunnel: w2155 -> [w2171 _ _ _ _ _ _ _ _ _]
              tunnel: w2145 -> [w2166 _ _ _ _ _ _ _ _ _]
              tunnel: w2154 -> [_ w2197 _ _ _ _ _ _ _ _]
              tunnel: w2153 -> [_ _ w2227 _ _ _ _ _ _ _]
              tunnel: w2152 -> [_ _ _ w2257 _ _ _ _ _ _]
              tunnel: w2151 -> [_ _ _ _ w2287 _ _ _ _ _]
              tunnel: w2150 -> [_ _ _ _ _ w2317 _ _ _ _]
              tunnel: w2149 -> [_ _ _ _ _ _ w2347 _ _ _]
              tunnel: w2148 -> [_ _ _ _ _ _ _ w2377 _ _]
              tunnel: w2147 -> [_ _ _ _ _ _ _ _ w2407 _]
              tunnel: w2146 -> [_ _ _ _ _ _ _ _ _ w2437]
              tunnel: w2144 -> [_ w2196 _ _ _ _ _ _ _ _]
              tunnel: w2143 -> [_ _ w2226 _ _ _ _ _ _ _]
              tunnel: w2142 -> [_ _ _ w2256 _ _ _ _ _ _]
              tunnel: w2141 -> [_ _ _ _ w2286 _ _ _ _ _]
              tunnel: w2140 -> [_ _ _ _ _ w2316 _ _ _ _]
              tunnel: w2139 -> [_ _ _ _ _ _ w2346 _ _ _]
              tunnel: w2138 -> [_ _ _ _ _ _ _ w2376 _ _]
              tunnel: w2137 -> [_ _ _ _ _ _ _ _ w2406 _]
              tunnel: w2136 -> [_ _ _ _ _ _ _ _ _ w2436]
              frame #0 {
                # "LAB01-1"
                n1191 = Equal?(x=w2171, y=2) -> (x = y?=w2169:bool)
                n1192 = local read "DISP LAB01-1"() -> (w2172:T4)
                n1193 = Unbundle(w2172) -> ("STATUS"=w2173:string)  [unwired: 2 out]
                n1194 = Equal?(x=w2173, y="RUN") -> (x = y?=w2168:bool)
                n1195 = And(x=w2168, y=w2169) -> (x .and. y?=w2167:bool)
